vi "UNITEST MAIN v2.0.vi"() -> ()   [LabVIEW 2025] (continued)
            n1370 = property on="Property Node" class="DigNum (strict)"(reference=w2222, "Minimum"=2.0 ("Data Entry Limits:Minimum"), "Maximum"=50.0 ("Data Entry Limits:Maximum"), "Increment"=0.1 ("Data Entry Limits:Increment")) -> (reference out=w2220:refnum<vi>, error out=w2221:errorcluster)  [unwired: 1 in]
            n1371 = call "DATA ENCRYPT STRING FILE WRITE.vi"("error in (no error)"=w2224, "User Action"="User selected 0.3 SSP", "main ref"=w2216) -> ("error out"=w2223:errorcluster)  [unwired: 6 in, 1 out]
            n1372 = Close Reference(reference=w2229, error in (no error)=w2228) -> ()  [unwired: 1 out]
            n1373 = Close Reference(reference=w2230, error in (no error)=w2231) -> ()  [unwired: 1 out]
            n1374 = Close Reference(reference=w2220, error in (no error)=w2221) -> ()  [unwired: 1 out]
          }
        }
      }
      frame "SSP 0.5" {
        n1375 = Unbundle By Name(w2235) -> ("Loading.SSP 0.5"=w2238:refnum<vi>)
        n1376 = property on="Property Node" class="Bool (strict)"(reference=w2238, error in=w2237) -> (reference out=w2240:refnum<vi>, error out=w2239:errorcluster, "Value"=w2236:bool)
        n1377 = Close Reference(reference=w2240, error in (no error)=w2239) -> (error out=w2234:errorcluster)
        n1378 = case shown="True" w2236 {
          tunnel: w2235 -> [_ w2242]
          tunnel: w2234 -> [w2241 w2250]
          tunnel: [w2241 w2249] -> w2233
          frame False {
          }
          frame True {
            w2252 = FALSE ("Value")
            n1379 = Unbundle By Name(w2242) -> ("Loading.Enter the Load  (N)"=w2248:refnum<vi>)
            n1380 = Unbundle By Name(w2242) -> ("Loading.SSP 0.75"=w2258:refnum<vi>)
            n1381 = Unbundle By Name(w2242) -> ("Loading.SSP 0.3"=w2253:refnum<vi>)
            n1382 = property on="Property Node" class="Bool (strict)"(reference=w2253, "Value"=w2252) -> (reference out=w2255:refnum<vi>, error out=w2254:errorcluster)  [unwired: 1 in]
            n1383 = property on="Property Node" class="Bool (strict)"(reference=w2258, "Value"=w2252) -> (reference out=w2256:refnum<vi>, error out=w2257:errorcluster)  [unwired: 1 in]
            n1384 = property on="Property Node" class="DigNum (strict)"(reference=w2248, "Minimum"=2.0 ("Data Entry Limits:Minimum"), "Maximum"=200.0 ("Data Entry Limits:Maximum"), "Increment"=0.1 ("Data Entry Limits:Increment")) -> (reference out=w2246:refnum<vi>, error out=w2247:errorcluster)  [unwired: 1 in]
            n1385 = call "DATA ENCRYPT STRING FILE WRITE.vi"("error in (no error)"=w2250, "User Action"="User selected 0.5 SSP", "main ref"=w2242) -> ("error out"=w2249:errorcluster)  [unwired: 6 in, 1 out]
            n1386 = Close Reference(reference=w2255, error in (no error)=w2254) -> ()  [unwired: 1 out]
            n1387 = Close Reference(reference=w2256, error in (no error)=w2257) -> ()  [unwired: 1 out]
            n1388 = Close Reference(reference=w2246, error in (no error)=w2247) -> ()  [unwired: 1 out]
          }
        }
      }
      frame "SSP 0.75" {
        n1389 = Unbundle By Name(w2261) -> ("Loading.SSP 0.75"=w2264:refnum<vi>)
        n1390 = property on="Property Node" class="Bool (strict)"(reference=w2264, error in=w2263) -> (reference out=w2266:refnum<vi>, error out=w2265:errorcluster, "Value"=w2262:bool)
        n1391 = Close Reference(reference=w2266, error in (no error)=w2265) -> (error out=w2260:errorcluster)
        n1392 = case shown="True" w2262 {
          tunnel: w2261 -> [_ w2268]
          tunnel: w2260 -> [w2267 w2276]
          tunnel: [w2267 w2275] -> w2259
          frame False {
          }
          frame True {
            w2278 = FALSE ("Value")
            n1393 = Unbundle By Name(w2268) -> ("Loading.SSP 0.3"=w2279:refnum<vi>)
            n1394 = Unbundle By Name(w2268) -> ("Loading.SSP 0.5"=w2284:refnum<vi>)
            n1395 = Unbundle By Name(w2268) -> ("Loading.Enter the Load  (N)"=w2274:refnum<vi>)
            n1396 = property on="Property Node" class="Bool (strict)"(reference=w2279, "Value"=w2278) -> (reference out=w2281:refnum<vi>, error out=w2280:errorcluster)  [unwired: 1 in]
            n1397 = property on="Property Node" class="Bool (strict)"(reference=w2284, "Value"=w2278) -> (reference out=w2282:refnum<vi>, error out=w2283:errorcluster)  [unwired: 1 in]
            n1398 = property on="Property Node" class="DigNum (strict)"(reference=w2274, "Minimum"=200.0 ("Data Entry Limits:Minimum"), "Maximum"=500.0 ("Data Entry Limits:Maximum"), "Increment"=0.1 ("Data Entry Limits:Increment")) -> (reference out=w2272:refnum<vi>, error out=w2273:errorcluster)  [unwired: 1 in]
            n1399 = call "DATA ENCRYPT STRING FILE WRITE.vi"("error in (no error)"=w2276, "User Action"="User selected 0.75 SSP", "main ref"=w2268) -> ("error out"=w2275:errorcluster)  [unwired: 6 in, 1 out]
            n1400 = Close Reference(reference=w2281, error in (no error)=w2280) -> ()  [unwired: 1 out]
            n1401 = Close Reference(reference=w2282, error in (no error)=w2283) -> ()  [unwired: 1 out]
            n1402 = Close Reference(reference=w2272, error in (no error)=w2273) -> ()  [unwired: 1 out]
          }
        }
      }
      frame "LHBack" {
        # "Back to Configure"
        n1403 = Unbundle By Name(w2286) -> ("Main Home Screen.GUI"=w2295:refnum<vi>)
        n1404 = Unbundle By Name(w2286) -> ("Main Home Screen.MainPage"=w2291:refnum<vi>)
        n1405 = Unbundle By Name(w2286) -> ("Loading.LHBack"=w2289:refnum<vi>)
        n1406 = property on="Property Node" class="TabCtl (strict)"(reference=w2291, "Value"=T16."HOME") -> (reference out=w2293:refnum<vi>, error out=w2292:errorcluster)  [unwired: 1 in]
        n1407 = property on="Property Node" class="Bool (strict)"(reference=w2289, "Value"=FALSE) -> (reference out=w2287:refnum<vi>, error out=w2288:errorcluster)  [unwired: 1 in]
        n1408 = property on="Property Node" class="TabCtl (strict)"(reference=w2295, "Value"=T15."Setup") -> (reference out=w2297:refnum<vi>, error out=w2296:errorcluster)  [unwired: 1 in]
        n1409 = Close Reference(reference=w2293, error in (no error)=w2292) -> ()  [unwired: 1 out]
        n1410 = Close Reference(reference=w2287, error in (no error)=w2288) -> ()  [unwired: 1 out]
        n1411 = Close Reference(reference=w2297, error in (no error)=w2296) -> ()  [unwired: 1 out]
        n1412 = call "DATA ENCRYPT STRING FILE WRITE.vi"("error in (no error)"=w2298, "User Action"="User selected Back to Configure", "main ref"=w2286) -> ("error out"=w2299:errorcluster)  [unwired: 6 in, 1 out]
      }
      frame "MMBack" {
        # "Back to Configure"
        n1413 = Unbundle By Name(w2301) -> ("Motion Module.MMBack"=w2305:refnum<vi>)
        n1414 = Unbundle By Name(w2301) -> ("Main Home Screen.GUI"=w2311:refnum<vi>)
        n1415 = Unbundle By Name(w2301) -> ("Main Home Screen.MainPage"=w2307:refnum<vi>)
        n1416 = property on="Property Node" class="Bool (strict)"(reference=w2305, "Value"=FALSE) -> (reference out=w2303:refnum<vi>, error out=w2304:errorcluster)  [unwired: 1 in]
        n1417 = property on="Property Node" class="TabCtl (strict)"(reference=w2307, "Value"=T16."HOME") -> (reference out=w2309:refnum<vi>, error out=w2308:errorcluster)  [unwired: 1 in]
        n1418 = property on="Property Node" class="TabCtl (strict)"(reference=w2311, "Value"=T15."Load Head") -> (reference out=w2313:refnum<vi>, error out=w2312:errorcluster)  [unwired: 1 in]
        n1419 = Close Reference(reference=w2303, error in (no error)=w2304) -> ()  [unwired: 1 out]
        n1420 = Close Reference(reference=w2309, error in (no error)=w2308) -> ()  [unwired: 1 out]
        n1421 = Close Reference(reference=w2313, error in (no error)=w2312) -> ()  [unwired: 1 out]
        n1422 = call "DATA ENCRYPT STRING FILE WRITE.vi"("error in (no error)"=w2314, "User Action"="User selected Back to Load Selection", "main ref"=w2301) -> ("error out"=w2315:errorcluster)  [unwired: 6 in, 1 out]
      }
      frame "LHNext" {
        w2351 = FALSE ("Visible")
        n1423 = Unbundle By Name(w2317) -> ("Motion Module.HomeRot"=w2357:refnum<vi>)
        n1424 = Unbundle By Name(w2317) -> ("Motion Module.HomeScratch"=w2352:refnum<vi>)
        n1425 = Unbundle By Name(w2317) -> ("Motion Module.PlaceModule"=w2350:refnum<vi>)
        n1426 = Unbundle By Name(w2317) -> ("Motion Module.Motion Mode:"=w2343:refnum<vi>)
        n1427 = Unbundle By Name(w2317) -> ("Motion Module.Motion Direction:  3"=w2342:refnum<vi>)
        n1428 = Unbundle By Name(w2317) -> ("Motion Module.Wear Track Diameter (mm)"=w2336:refnum<vi>)
        n1429 = Unbundle By Name(w2317) -> ("Motion Module.Set WTD"=w2333:refnum<vi>)
        n1430 = Unbundle By Name(w2317) -> ("Motion Module.Rotary Module Selection"=w2327:refnum<vi>)
        n1431 = call "DATA ENCRYPT STRING FILE WRITE.vi"("error in (no error)"=w2366, "User Action"="User selected Select Module", "main ref"=w2317) -> ("error out"=w2330:errorcluster)  [unwired: 6 in, 1 out]
        n1432 = property on="Property Node" class="TabCtl (strict)"(reference=w2327, "Visible"=FALSE) -> (reference out=w2326:refnum<vi>, error out=w2328:errorcluster)  [unwired: 1 in]
        n1433 = property on="Property Node" class="Bool (strict)"(reference=w2357, error in=w2330, "Visible"=w2351) -> (reference out=w2355:refnum<vi>, error out=w2356:errorcluster)
        n1434 = property on="Property Node" class="Bool (strict)"(reference=w2352, error in=w2330, "Visible"=w2351) -> (reference out=w2354:refnum<vi>, error out=w2353:errorcluster)
        n1435 = property on="Property Node" class="Bool (strict)"(reference=w2350, error in=w2330, "Visible"=TRUE) -> (reference out=w2348:refnum<vi>, error out=w2349:errorcluster)
        n1436 = property on="Property Node" class="Ring (strict)"(reference=w2343, error in=w2330, "Visible"=FALSE) -> (reference out=w2345:refnum<vi>, error out=w2344:errorcluster)
        n1437 = property on="Property Node" class="Ring (strict)"(reference=w2342, error in=w2330, "Visible"=FALSE) -> (reference out=w2339:refnum<vi>, error out=w2341:errorcluster)
        n1438 = property on="Property Node" class="DigNum (strict)"(reference=w2336, "Visible"=FALSE) -> (reference out=w2335:refnum<vi>, error out=w2337:errorcluster)  [unwired: 1 in]
        n1439 = property on="Property Node" class="Bool (strict)"(reference=w2333, "Visible"=FALSE) -> (reference out=w2334:refnum<vi>, error out=w2332:errorcluster)  [unwired: 1 in]
        n1440 = Close Reference(reference=w2355, error in (no error)=w2356) -> ()  [unwired: 1 out]
        n1441 = Close Reference(reference=w2354, error in (no error)=w2353) -> ()  [unwired: 1 out]
        n1442 = Close Reference(reference=w2348, error in (no error)=w2349) -> ()  [unwired: 1 out]
        n1443 = Close Reference(reference=w2345, error in (no error)=w2344) -> ()  [unwired: 1 out]
        n1444 = Close Reference(reference=w2339, error in (no error)=w2341) -> ()  [unwired: 1 out]
        n1445 = Close Reference(reference=w2335, error in (no error)=w2337) -> ()  [unwired: 1 out]
        n1446 = Close Reference(reference=w2326, error in (no error)=w2328) -> ()  [unwired: 1 out]
        n1447 = Close Reference(reference=w2334, error in (no error)=w2332) -> ()  [unwired: 1 out]
        n1448 = Unbundle By Name(w2317) -> ("Motion Module.M3 Image"=w2325:refnum<vi>)
        n1449 = Unbundle By Name(w2317) -> ("Main Home Screen.GUI"=w2363:refnum<vi>)
        n1450 = Unbundle By Name(w2317) -> ("Main Home Screen.MainPage"=w2359:refnum<vi>)
        n1451 = Unbundle By Name(w2317) -> ("Loading.LHNext"=w2321:refnum<vi>)
        n1452 = property on="Property Node" class="TabCtl (strict)"(reference=w2325, "Value"=enum32{"Page 1", "Page 2"}."Page 2") -> (reference out=w2323:refnum<vi>, error out=w2324:errorcluster)  [unwired: 1 in]
        n1453 = property on="Property Node" class="TabCtl (strict)"(reference=w2359, "Value"=T16."HOME") -> (reference out=w2361:refnum<vi>, error out=w2360:errorcluster)  [unwired: 1 in]
        n1454 = property on="Property Node" class="TabCtl (strict)"(reference=w2363, "Value"=T15."Motion Module") -> (reference out=w2365:refnum<vi>, error out=w2364:errorcluster)  [unwired: 1 in]
        n1455 = property on="Property Node" class="Bool (strict)"(reference=w2321, "Value"=FALSE ("Visible")) -> (reference out=w2318:refnum<vi>, error out=w2320:errorcluster)  [unwired: 1 in]
        n1456 = Close Reference(reference=w2323, error in (no error)=w2324) -> ()  [unwired: 1 out]
        n1457 = Close Reference(reference=w2318, error in (no error)=w2320) -> ()  [unwired: 1 out]
        n1458 = Close Reference(reference=w2361, error in (no error)=w2360) -> ()  [unwired: 1 out]
        n1459 = Close Reference(reference=w2365, error in (no error)=w2364) -> ()  [unwired: 1 out]
      }
      frame "Rot Ver" {
        n1460 = call "Rotory Module Selection.vi"("error in (no error)"=w2370, "Data Cluster"=w2368) -> ("error out"=w2369:errorcluster)  [unwired: 9 in]
      }
      frame "Scratch" {
        n1461 = call "Scratch Module Selection.vi"("error in (no error)"=w2373, "Data Cluster"=w2371) -> ("error out"=w2372:errorcluster)  [unwired: 9 in]
      }
      frame "Traction" {
        n1462 = call "TractionModule Selection.vi"("error in (no error)"=w2376, "Data Cluster"=w2374) -> ("error out"=w2375:errorcluster)  [unwired: 9 in]
      }
      frame "Motion Mode:" {
        n1463 = Unbundle By Name(w2377) -> ("Motion Module.Motion Mode:"=w2379:refnum<vi>)
        n1464 = property on="Property Node" class="Ring (strict)"(reference=w2379) -> (reference out=w2381:refnum<vi>, error out=w2380:errorcluster, "Value"=w2378:u16)  [unwired: 1 in]
        n1465 = Close Reference(reference=w2381, error in (no error)=w2380) -> ()  [unwired: 1 out]
        n1466 = case shown="3" w2378 {
          tunnel: w2383 -> [w2400 w2417 w2434 w2451]
          tunnel: [w2399 w2416 w2433 w2450] -> w2382
          tunnel: w2377 -> [w2398 w2415 w2432 w2449]
          tunnel: w2377 -> [w2384 w2402 w2418 w2435]
          frame 0, Default {
            n1467 = Unbundle By Name(w2384) -> ("Motion Module.Rotary Module Selection"=w2394:refnum<vi>)
            n1468 = Unbundle By Name(w2384) -> ("Motion Module.Motion Direction:  3"=w2392:refnum<vi>)
            n1469 = Unbundle By Name(w2384) -> ("Main Screen.Angle (Deg)"=w2386:refnum<vi>)
            n1470 = property on="Property Node" class="TabCtl (strict)"(reference=w2394, "Value"=T18."Uniform Rotation") -> (reference out=w2396:refnum<vi>, error out=w2395:errorcluster)  [unwired: 1 in]
            n1471 = property on="Property Node" class="DigNum (strict)"(reference=w2386, "DisabledEnum"=T31."Disabled and Grayed Out" ("Disabled")) -> (reference out=w2388:refnum<vi>, error out=w2387:errorcluster)  [unwired: 1 in]
            n1472 = property on="Property Node" class="Ring (strict)"(reference=w2392, "Visible"=TRUE) -> (reference out=w2390:refnum<vi>, error out=w2391:errorcluster)  [unwired: 1 in]
            n1473 = Close Reference(reference=w2396, error in (no error)=w2395) -> ()  [unwired: 1 out]
            n1474 = Close Reference(reference=w2388, error in (no error)=w2387) -> ()  [unwired: 1 out]
            n1475 = Close Reference(reference=w2390, error in (no error)=w2391) -> ()  [unwired: 1 out]
            n1476 = call "DATA ENCRYPT STRING FILE WRITE.vi"("error in (no error)"=w2400, "User Action"="User Selected Uniform Rotation", "main ref"=w2398) -> ("error out"=w2399:errorcluster)  [unwired: 6 in, 1 out]
          }
          frame 1 {
            n1477 = Unbundle By Name(w2402) -> ("Motion Module.Rotary Module Selection"=w2411:refnum<vi>)
            n1478 = Unbundle By Name(w2402) -> ("Motion Module.Motion Direction:  3"=w2409:refnum<vi>)
            n1479 = Unbundle By Name(w2402) -> ("Main Screen.Angle (Deg)"=w2403:refnum<vi>)
            n1480 = property on="Property Node" class="TabCtl (strict)"(reference=w2411, "Value"=T18."Angular Oscillation") -> (reference out=w2413:refnum<vi>, error out=w2412:errorcluster)  [unwired: 1 in]
            n1481 = property on="Property Node" class="DigNum (strict)"(reference=w2403, "DisabledEnum"=T31."Enabled" ("Disabled")) -> (reference out=w2405:refnum<vi>, error out=w2404:errorcluster)  [unwired: 1 in]
            n1482 = property on="Property Node" class="Ring (strict)"(reference=w2409, "Visible"=FALSE) -> (reference out=w2407:refnum<vi>, error out=w2408:errorcluster)  [unwired: 1 in]
            n1483 = Close Reference(reference=w2413, error in (no error)=w2412) -> ()  [unwired: 1 out]
            n1484 = Close Reference(reference=w2407, error in (no error)=w2408) -> ()  [unwired: 1 out]
            n1485 = Close Reference(reference=w2405, error in (no error)=w2404) -> ()  [unwired: 1 out]
            n1486 = call "DATA ENCRYPT STRING FILE WRITE.vi"("error in (no error)"=w2417, "User Action"="User Selected Angular Oscillation", "main ref"=w2415) -> ("error out"=w2416:errorcluster)  [unwired: 6 in, 1 out]
          }
          frame 2 {
            n1487 = Unbundle By Name(w2418) -> ("Motion Module.Rotary Module Selection"=w2428:refnum<vi>)
            n1488 = Unbundle By Name(w2418) -> ("Motion Module.Motion Direction:  3"=w2426:refnum<vi>)
            n1489 = Unbundle By Name(w2418) -> ("Main Screen.Angle (Deg)"=w2420:refnum<vi>)
            n1490 = property on="Property Node" class="DigNum (strict)"(reference=w2420, "DisabledEnum"=T31."Disabled and Grayed Out" ("Disabled")) -> (reference out=w2422:refnum<vi>, error out=w2421:errorcluster)  [unwired: 1 in]
            n1491 = property on="Property Node" class="TabCtl (strict)"(reference=w2428, "Value"=T18."Speed Ramp") -> (reference out=w2430:refnum<vi>, error out=w2429:errorcluster)  [unwired: 1 in]
            n1492 = property on="Property Node" class="Ring (strict)"(reference=w2426, "Visible"=TRUE) -> (reference out=w2424:refnum<vi>, error out=w2425:errorcluster)  [unwired: 1 in]
            n1493 = Close Reference(reference=w2422, error in (no error)=w2421) -> ()  [unwired: 1 out]
            n1494 = Close Reference(reference=w2430, error in (no error)=w2429) -> ()  [unwired: 1 out]
            n1495 = Close Reference(reference=w2424, error in (no error)=w2425) -> ()  [unwired: 1 out]
            n1496 = call "DATA ENCRYPT STRING FILE WRITE.vi"("error in (no error)"=w2434, "User Action"="User Selected Ramp Mode", "main ref"=w2432) -> ("error out"=w2433:errorcluster)  [unwired: 6 in, 1 out]
          }
          frame 3 {
            n1497 = Unbundle By Name(w2435) -> ("Motion Module.Rotary Module Selection"=w2445:refnum<vi>)
            n1498 = Unbundle By Name(w2435) -> ("Motion Module.Motion Direction:  3"=w2443:refnum<vi>)
            n1499 = Unbundle By Name(w2435) -> ("Main Screen.Angle (Deg)"=w2437:refnum<vi>)
            n1500 = property on="Property Node" class="TabCtl (strict)"(reference=w2445, "Value"=T18."Speed Step") -> (reference out=w2447:refnum<vi>, error out=w2446:errorcluster)  [unwired: 1 in]
            n1501 = property on="Property Node" class="DigNum (strict)"(reference=w2437, "DisabledEnum"=T31."Disabled and Grayed Out" ("Disabled")) -> (reference out=w2439:refnum<vi>, error out=w2438:errorcluster)  [unwired: 1 in]
            n1502 = property on="Property Node" class="Ring (strict)"(reference=w2443, "Visible"=FALSE) -> (reference out=w2441:refnum<vi>, error out=w2442:errorcluster)  [unwired: 1 in]
            n1503 = Close Reference(reference=w2447, error in (no error)=w2446) -> ()  [unwired: 1 out]
            n1504 = Close Reference(reference=w2439, error in (no error)=w2438) -> ()  [unwired: 1 out]
            n1505 = Close Reference(reference=w2441, error in (no error)=w2442) -> ()  [unwired: 1 out]
            n1506 = call "DATA ENCRYPT STRING FILE WRITE.vi"("error in (no error)"=w2451, "User Action"="User Selected Step Mode", "main ref"=w2449) -> ("error out"=w2450:errorcluster)  [unwired: 6 in, 1 out]
          }
        }
      }
      frame "MMNext" {
        n1507 = Unbundle By Name(w2452) -> ("Motion Module.MMNext"=w2457:refnum<vi>)
        n1508 = Unbundle By Name(w2452) -> ("Motion Module.MMNext"=w2464:refnum<vi>)
        n1509 = Unbundle By Name(w2452) -> ("Main Home Screen.GUI"=w2466:refnum<vi>)
        n1510 = property on="Property Node" class="Bool (strict)"(reference=w2457, "Value"=FALSE ("Visible")) -> (reference out=w2454:refnum<vi>, error out=w2456:errorcluster)  [unwired: 1 in]
        n1511 = property on="Property Node" class="TabCtl (strict)"(reference=w2466, "Value"=T15."Environment") -> (reference out=w2468:refnum<vi>, error out=w2467:errorcluster)  [unwired: 1 in]
        n1512 = property on="Property Node" class="Bool (strict)"(reference=w2464, "Value"=FALSE) -> (reference out=w2462:refnum<vi>, error out=w2463:errorcluster)  [unwired: 1 in]
        n1513 = Close Reference(reference=w2454, error in (no error)=w2456) -> ()  [unwired: 1 out]
        n1514 = Close Reference(reference=w2462, error in (no error)=w2463) -> ()  [unwired: 1 out]
        n1515 = Close Reference(reference=w2468, error in (no error)=w2467) -> ()  [unwired: 1 out]
        n1516 = call "DATA ENCRYPT STRING FILE WRITE.vi"("error in (no error)"=w2459, "User Action"="User Selected SetUp Module", "main ref"=w2452) -> ("error out"=w2458:errorcluster)  [unwired: 6 in, 1 out]
        n1517 = call "Main Screen Tab Visible.vi"("error in (no error)"=w2458, "main ref"=w2452) -> ("error out"=w2453:errorcluster)  [unwired: 9 in]
      }
      frame "APBack" {
        n1518 = Unbundle By Name(w2469) -> ("Environmental control.APBack"=w2476:refnum<vi>)
        n1519 = Unbundle By Name(w2469) -> ("Main Home Screen.GUI"=w2478:refnum<vi>)
        n1520 = property on="Property Node" class="TabCtl (strict)"(reference=w2478, "Value"=T15."Motion Module") -> (reference out=w2480:refnum<vi>, error out=w2479:errorcluster)  [unwired: 1 in]
        n1521 = property on="Property Node" class="Bool (strict)"(reference=w2476, "Value"=FALSE) -> (reference out=w2474:refnum<vi>, error out=w2475:errorcluster)  [unwired: 1 in]
        n1522 = Close Reference(reference=w2474, error in (no error)=w2475) -> ()  [unwired: 1 out]
        n1523 = Close Reference(reference=w2480, error in (no error)=w2479) -> ()  [unwired: 1 out]
        n1524 = call "DATA ENCRYPT STRING FILE WRITE.vi"("error in (no error)"=w2471, "User Action"="User Selected Back to Module", "main ref"=w2469) -> ("error out"=w2470:errorcluster)  [unwired: 6 in, 1 out]
      }
      frame "SNext" {
        n1525 = Unbundle By Name(w2482) -> ("Environmental control.Acoustic Emission 3"=w2486:refnum<vi>)
        n1526 = property on="Property Node" class="Bool (strict)"(reference=w2486) -> (reference out=w2484:refnum<vi>, error out=w2485:errorcluster, "Value"=w2481:bool)  [unwired: 1 in]
        n1527 = Close Reference(reference=w2484, error in (no error)=w2485) -> ()  [unwired: 1 out]
        n1528 = case shown="True" w2481 {
          tunnel: w2488 -> [w2491 w2495]
          tunnel: [w2491 w2492] -> w2483
          tunnel: w2482 -> [_ w2493]
          frame False {
          }
          frame True {
            n1529 = call "Acq Gain Selection.vi"("error in (no error)"=w2495, "Data Cluster"=w2493) -> ("error out"=w2494:errorcluster)  [unwired: 9 in]
            n1530 = call <vilib>:"Clear Errors.vi"("error in (no error)"=w2494) -> ("error out"=w2492:errorcluster)  [unwired: 5 in, 1 out]
          }
        }
        n1531 = call "Init Before Main Screen.vi"("error in (no error)"=w2483, "Data Cluster"=w2482) -> ("error out"=w2487:errorcluster)  [unwired: 9 in]
        n1532 = call "DATA ENCRYPT STRING FILE WRITE.vi"("error in (no error)"=w2487, "User Action"="User Pressed Setup", "main ref"=w2482) -> ("error out"=w2489:errorcluster)  [unwired: 6 in, 1 out]
      }
      frame "Enable Platform" {
        n1533 = call "Reinitialise Load cell after Error.vi"("error in (no error)"=w2499, "main ref"=w2496) -> ("error out"=w2497:errorcluster)  [unwired: 9 in]
        n1534 = Unbundle By Name(w2496) -> ("Platform Settings.Enable Platform"=w2523:refnum<vi>)
        n1535 = Bundle By Name(cluster=T9 {"Sequence ID"=0, "Mode Command"=0, "Distance"=0.0, "SPEED"=0.0, "Reserved"=0.0, "SPARE 1"=0, "SPARE 2"=0, "SPARE 3"=0, "SPARE 4"=0, "SPARE 5"=0, "SPARE 6"=0, "SPARE 7"=0, "SPARE 8"=0, "SPARE 9"=0, "SPARE 10"=0, "SPARE 11"=0, "SPARE 12"=0, "SPARE 13"=0, "SPARE 14"=0, "SPARE 15"=0, "SPARE 16"=0, "SPARE 17"=0} ("Value"), "Mode Command"=u8 1, "Distance"=sgl 0.0, "SPEED"=sgl 0.0, "Sequence ID"=u16 0) -> (w2508:T9)
        n1536 = Unbundle By Name(w2496) -> ("Heave AND Surge.UPLINK HEAVE"=w2501:refnum<vi>)
        n1537 = property on="Property Node" class="Bool (strict)"(reference=w2523, "Value"=FALSE) -> (reference out=w2521:refnum<vi>, error out=w2522:errorcluster)  [unwired: 1 in]
        n1538 = property on="Property Node" class="Clust (strict)"(reference=w2501, error in=w2497, "Value"=w2508) -> (reference out=w2507:refnum<vi>, error out=w2506:errorcluster)
        n1539 = Close Reference(reference=w2521, error in (no error)=w2522) -> ()  [unwired: 1 out]
        n1540 = Close Reference(reference=w2507, error in (no error)=w2506) -> (error out=w2498:errorcluster)
        n1541 = call "DATA ENCRYPT STRING FILE WRITE.vi"("error in (no error)"=w2498, "User Action"="User Pressed Enable Platform", "main ref"=w2496) -> ("error out"=w2510:errorcluster)  [unwired: 6 in, 1 out]
        n1542 = call "HEAVE WRITE FGV.vi"("Enum - Menu"=Heave_Write_enum."WRITE", "error in (no error)"=w2510, "main ref"=w2496) -> ("error out"=w2513:errorcluster)  [unwired: 8 in]
        n1543 = call "TRACTION HOME.vi"("error in (no error)"=w2510, "Data Cluster"=w2496) -> ("error out"=→"error out":errorcluster)  [unwired: 9 in]
        n1544 = Unbundle By Name(w2496) -> ("Heave AND Surge.Read Heave Temp"=w2517:refnum<vi>)
        n1545 = property on="Property Node" class="Bool (strict)"(reference=w2517, error in=w2513, "Value"=TRUE) -> (reference out=w2515:refnum<vi>, error out=w2516:errorcluster)
        n1546 = Close Reference(reference=w2515, error in (no error)=w2516) -> (error out=w2512:errorcluster)
        "HEAVE ENABLE" <- TRUE ("HEAVE ENABLE")
      }
      frame "Heave Up main" {
        n1547 = Unbundle By Name(w2524) -> ("Platform Settings.Heave Up main"=w2534:refnum<vi>)
        n1548 = call "Heave Up Main.vi"("error in (no error)"=w2526, "main ref"=w2524) -> ("error out"=w2525:errorcluster)  [unwired: 9 in]
        n1549 = property on="Property Node" class="Bool (strict)"(reference=w2534, "Value"=FALSE) -> (reference out=w2532:refnum<vi>, error out=w2533:errorcluster)  [unwired: 1 in]
        n1550 = Close Reference(reference=w2532, error in (no error)=w2533) -> ()  [unwired: 1 out]
        n1551 = call "DATA ENCRYPT STRING FILE WRITE.vi"("error in (no error)"=w2525, "User Action"="User Pressed Heave UP", "main ref"=w2524) -> ("error out"=w2529:errorcluster)  [unwired: 6 in, 1 out]
        n1552 = call "HEAVE WRITE FGV.vi"("Enum - Menu"=Heave_Write_enum."WRITE", "error in (no error)"=w2529, "main ref"=w2524) -> ("error out"=w2528:errorcluster)  [unwired: 8 in]
      }
      frame "Heave Up MM" {
        n1553 = Unbundle By Name(w2535) -> ("Motion Module.Heave Up MM"=w2545:refnum<vi>)
        n1554 = call "Heave Up Motion Module.vi"("error in (no error)"=w2537, "main ref"=w2535) -> ("error out"=w2536:errorcluster)  [unwired: 9 in]
        n1555 = property on="Property Node" class="Bool (strict)"(reference=w2545, "Value"=FALSE) -> (reference out=w2543:refnum<vi>, error out=w2544:errorcluster)  [unwired: 1 in]
        n1556 = Close Reference(reference=w2543, error in (no error)=w2544) -> ()  [unwired: 1 out]
        n1557 = call "DATA ENCRYPT STRING FILE WRITE.vi"("error in (no error)"=w2536, "User Action"="User Pressed Heave UP in Motion Module", "main ref"=w2535) -> ("error out"=w2540:errorcluster)  [unwired: 6 in, 1 out]
        n1558 = call "HEAVE WRITE FGV.vi"("Enum - Menu"=Heave_Write_enum."WRITE", "error in (no error)"=w2540, "main ref"=w2535) -> ("error out"=w2539:errorcluster)  [unwired: 8 in]
      }
      frame "Heave Down Main" {
        n1559 = call "Heave Down Main.vi"("error in (no error)"=w2548, "main ref"=w2546) -> ("error out"=w2547:errorcluster)  [unwired: 9 in]
        n1560 = Unbundle By Name(w2546) -> ("Platform Settings.Heave Down Main"=w2556:refnum<vi>)
        n1561 = property on="Property Node" class="Bool (strict)"(reference=w2556, "Value"=FALSE) -> (reference out=w2554:refnum<vi>, error out=w2555:errorcluster)  [unwired: 1 in]
        n1562 = Close Reference(reference=w2554, error in (no error)=w2555) -> ()  [unwired: 1 out]
        n1563 = call "DATA ENCRYPT STRING FILE WRITE.vi"("error in (no error)"=w2547, "User Action"="User Pressed Heave DOWN", "main ref"=w2546) -> ("error out"=w2551:errorcluster)  [unwired: 6 in, 1 out]
        n1564 = call "HEAVE WRITE FGV.vi"("Enum - Menu"=Heave_Write_enum."WRITE", "error in (no error)"=w2551, "main ref"=w2546) -> ("error out"=w2550:errorcluster)  [unwired: 8 in]
      }
      frame "Heave Down MM" {
        n1565 = call "Heave Down Motion Module.vi"("error in (no error)"=w2559, "main ref"=w2557) -> ("error out"=w2558:errorcluster)  [unwired: 9 in]
        n1566 = Unbundle By Name(w2557) -> ("Motion Module.Heave Down MM"=w2567:refnum<vi>)
        n1567 = property on="Property Node" class="Bool (strict)"(reference=w2567, "Value"=FALSE) -> (reference out=w2565:refnum<vi>, error out=w2566:errorcluster)  [unwired: 1 in]
        n1568 = Close Reference(reference=w2565, error in (no error)=w2566) -> ()  [unwired: 1 out]
        n1569 = call "DATA ENCRYPT STRING FILE WRITE.vi"("error in (no error)"=w2558, "User Action"="User Pressed Heave DOWN in Motion Module", "main ref"=w2557) -> ("error out"=w2562:errorcluster)  [unwired: 6 in, 1 out]
        n1570 = call "HEAVE WRITE FGV.vi"("Enum - Menu"=Heave_Write_enum."WRITE", "error in (no error)"=w2562, "main ref"=w2557) -> ("error out"=w2561:errorcluster)  [unwired: 8 in]
      }
      frame "Surge Backward Main" {
        n1571 = Unbundle By Name(w2568) -> ("Platform Settings.Surge Backward Main"=w2578:refnum<vi>)
        n1572 = call "Surge Backward Main.vi"("error in (no error)"=w2570, "main ref"=w2568) -> ("error out"=w2569:errorcluster)  [unwired: 9 in]
        n1573 = property on="Property Node" class="Bool (strict)"(reference=w2578, "Value"=FALSE) -> (reference out=w2576:refnum<vi>, error out=w2577:errorcluster)  [unwired: 1 in]
        n1574 = Close Reference(reference=w2576, error in (no error)=w2577) -> ()  [unwired: 1 out]
        n1575 = call "DATA ENCRYPT STRING FILE WRITE.vi"("error in (no error)"=w2569, "User Action"="User Pressed Surge Backward", "main ref"=w2568) -> ("error out"=w2573:errorcluster)  [unwired: 6 in, 1 out]
        n1576 = call "HEAVE WRITE FGV.vi"("Enum - Menu"=Heave_Write_enum."WRITE", "error in (no error)"=w2573, "main ref"=w2568) -> ("error out"=w2572:errorcluster)  [unwired: 8 in]
      }
      frame "Surge Backward MM" {
        n1577 = Unbundle By Name(w2579) -> ("Motion Module.Surge Backward MM"=w2589:refnum<vi>)
        n1578 = call "Surge Backward MM.vi"("error in (no error)"=w2581, "main ref"=w2579) -> ("error out"=w2580:errorcluster)  [unwired: 9 in]
        n1579 = property on="Property Node" class="Bool (strict)"(reference=w2589, "Value"=FALSE) -> (reference out=w2587:refnum<vi>, error out=w2588:errorcluster)  [unwired: 1 in]
        n1580 = Close Reference(reference=w2587, error in (no error)=w2588) -> ()  [unwired: 1 out]
        n1581 = call "DATA ENCRYPT STRING FILE WRITE.vi"("error in (no error)"=w2580, "User Action"="User Pressed Surge Backward in Motion Module", "main ref"=w2579) -> ("error out"=w2584:errorcluster)  [unwired: 6 in, 1 out]
        n1582 = call "HEAVE WRITE FGV.vi"("Enum - Menu"=Heave_Write_enum."WRITE", "error in (no error)"=w2584, "main ref"=w2579) -> ("error out"=w2583:errorcluster)  [unwired: 8 in]
      }
      frame "Surge Forward Main" {
        n1583 = Unbundle By Name(w2590) -> ("Platform Settings.Surge Forward Main"=w2600:refnum<vi>)
        n1584 = call "Surge Forward Main.vi"("error in (no error)"=w2592, "main ref"=w2590) -> ("error out"=w2591:errorcluster)  [unwired: 9 in]
        n1585 = property on="Property Node" class="Bool (strict)"(reference=w2600, "Value"=FALSE) -> (reference out=w2598:refnum<vi>, error out=w2599:errorcluster)  [unwired: 1 in]
        n1586 = Close Reference(reference=w2598, error in (no error)=w2599) -> ()  [unwired: 1 out]
        n1587 = call "DATA ENCRYPT STRING FILE WRITE.vi"("error in (no error)"=w2591, "User Action"="User Pressed Surge Forward", "main ref"=w2590) -> ("error out"=w2595:errorcluster)  [unwired: 6 in, 1 out]
        n1588 = call "HEAVE WRITE FGV.vi"("Enum - Menu"=Heave_Write_enum."WRITE", "error in (no error)"=w2595, "main ref"=w2590) -> ("error out"=w2594:errorcluster)  [unwired: 8 in]
      }
      frame "Surge Forward MM" {
        n1589 = Unbundle By Name(w2601) -> ("Motion Module.Surge Forward MM"=w2611:refnum<vi>)
        n1590 = call "Surge Forward MM.vi"("error in (no error)"=w2603, "main ref"=w2601) -> ("error out"=w2602:errorcluster)  [unwired: 9 in]
        n1591 = property on="Property Node" class="Bool (strict)"(reference=w2611, "Value"=FALSE) -> (reference out=w2609:refnum<vi>, error out=w2610:errorcluster)  [unwired: 1 in]
        n1592 = Close Reference(reference=w2609, error in (no error)=w2610) -> ()  [unwired: 1 out]
        n1593 = call "DATA ENCRYPT STRING FILE WRITE.vi"("error in (no error)"=w2602, "User Action"="User Pressed Surge Forward in Motion Module", "main ref"=w2601) -> ("error out"=w2606:errorcluster)  [unwired: 6 in, 1 out]
        n1594 = call "HEAVE WRITE FGV.vi"("Enum - Menu"=Heave_Write_enum."WRITE", "error in (no error)"=w2606, "main ref"=w2601) -> ("error out"=w2605:errorcluster)  [unwired: 8 in]
      }
      frame "Sway Left Main" {
        n1595 = call "Sway Left Main.vi"("error in (no error)"=w2615, "main ref"=w2613) -> ("error out"=w2614:errorcluster)  [unwired: 9 in]
        n1596 = Unbundle By Name(w2613) -> ("Platform Settings.Sway Left Main"=w2622:refnum<vi>)
        n1597 = property on="Property Node" class="Bool (strict)"(reference=w2622, "Value"=FALSE) -> (reference out=w2620:refnum<vi>, error out=w2621:errorcluster)  [unwired: 1 in]
        n1598 = Close Reference(reference=w2620, error in (no error)=w2621) -> ()  [unwired: 1 out]
        n1599 = call "DATA ENCRYPT STRING FILE WRITE.vi"("error in (no error)"=w2614, "User Action"="User Pressed Sway Left ", "main ref"=w2613) -> ("error out"=w2617:errorcluster)  [unwired: 6 in, 1 out]
        n1600 = call "SWAY WRITE FGV.vi"("Enum - Menu"=Sway_Write_enum."WRITE", "error in (no error)"=w2617, "main ref"=w2613) -> ("error out"=w2616:errorcluster)  [unwired: 8 in]
      }
      frame "Sway Left MM" {
        n1601 = call "Sway Left MM.vi"("error in (no error)"=w2626, "main ref"=w2624) -> ("error out"=w2625:errorcluster)  [unwired: 9 in]
        n1602 = Unbundle By Name(w2624) -> ("Motion Module.Sway Left MM"=w2633:refnum<vi>)
        n1603 = property on="Property Node" class="Bool (strict)"(reference=w2633, "Value"=FALSE) -> (reference out=w2631:refnum<vi>, error out=w2632:errorcluster)  [unwired: 1 in]
        n1604 = Close Reference(reference=w2631, error in (no error)=w2632) -> ()  [unwired: 1 out]
        n1605 = call "DATA ENCRYPT STRING FILE WRITE.vi"("error in (no error)"=w2625, "User Action"="User Pressed Sway Left in MM", "main ref"=w2624) -> ("error out"=w2628:errorcluster)  [unwired: 6 in, 1 out]
        n1606 = call "SWAY WRITE FGV.vi"("Enum - Menu"=Sway_Write_enum."WRITE", "error in (no error)"=w2628, "main ref"=w2624) -> ("error out"=w2627:errorcluster)  [unwired: 8 in]
      }
      frame "Sway Right MM" {
        n1607 = call "Sway Right MM.vi"("error in (no error)"=w2637, "main ref"=w2635) -> ("error out"=w2636:errorcluster)  [unwired: 9 in]
        n1608 = Unbundle By Name(w2635) -> ("Motion Module.Sway Right MM"=w2644:refnum<vi>)
        n1609 = property on="Property Node" class="Bool (strict)"(reference=w2644, "Value"=FALSE) -> (reference out=w2642:refnum<vi>, error out=w2643:errorcluster)  [unwired: 1 in]
        n1610 = Close Reference(reference=w2642, error in (no error)=w2643) -> ()  [unwired: 1 out]
        n1611 = call "DATA ENCRYPT STRING FILE WRITE.vi"("error in (no error)"=w2636, "User Action"="User Pressed Sway Right in MM", "main ref"=w2635) -> ("error out"=w2639:errorcluster)  [unwired: 6 in, 1 out]
        n1612 = call "SWAY WRITE FGV.vi"("Enum - Menu"=Sway_Write_enum."WRITE", "error in (no error)"=w2639, "main ref"=w2635) -> ("error out"=w2638:errorcluster)  [unwired: 8 in]
      }
      frame "Sway Right Main" {
        n1613 = call "Sway Right Main.vi"("error in (no error)"=w2648, "main ref"=w2646) -> ("error out"=w2647:errorcluster)  [unwired: 9 in]
        n1614 = Unbundle By Name(w2646) -> ("Platform Settings.Sway Right Main"=w2655:refnum<vi>)
        n1615 = property on="Property Node" class="Bool (strict)"(reference=w2655, "Value"=FALSE) -> (reference out=w2653:refnum<vi>, error out=w2654:errorcluster)  [unwired: 1 in]
        n1616 = Close Reference(reference=w2653, error in (no error)=w2654) -> ()  [unwired: 1 out]
        n1617 = call "DATA ENCRYPT STRING FILE WRITE.vi"("error in (no error)"=w2647, "User Action"="User Pressed Sway Right", "main ref"=w2646) -> ("error out"=w2650:errorcluster)  [unwired: 6 in, 1 out]
        n1618 = call "SWAY WRITE FGV.vi"("Enum - Menu"=Sway_Write_enum."WRITE", "error in (no error)"=w2650, "main ref"=w2646) -> ("error out"=w2649:errorcluster)  [unwired: 8 in]
      }
      frame "Manual Write Heave & Surge" {
        n1619 = Unbundle By Name(w2656) -> ("Heave AND Surge.Manual Write"=w2665:refnum<vi>)
        n1620 = property on="Property Node" class="Bool (strict)"(reference=w2665, "Value"=FALSE) -> (reference out=w2663:refnum<vi>, error out=w2664:errorcluster)  [unwired: 1 in]
        n1621 = Close Reference(reference=w2663, error in (no error)=w2664) -> ()  [unwired: 1 out]
        n1622 = call "DATA ENCRYPT STRING FILE WRITE.vi"("error in (no error)"=w2657, "User Action"="User Pressed Manual Write Heave and Surge", "main ref"=w2656) -> ("error out"=w2660:errorcluster)  [unwired: 6 in, 1 out]
        n1623 = call "HEAVE WRITE FGV.vi"("Enum - Menu"=Heave_Write_enum."WRITE", "error in (no error)"=w2660, "main ref"=w2656) -> ("error out"=w2659:errorcluster)  [unwired: 8 in]
      }
      frame "Manual Write SWAY" {
        n1624 = Unbundle By Name(w2667) -> ("SWAY.Manual Write SWAY"=w2675:refnum<vi>)
        n1625 = property on="Property Node" class="Bool (strict)"(reference=w2675, "Value"=FALSE) -> (reference out=w2673:refnum<vi>, error out=w2674:errorcluster)  [unwired: 1 in]
        n1626 = Close Reference(reference=w2673, error in (no error)=w2674) -> ()  [unwired: 1 out]
        n1627 = call "DATA ENCRYPT STRING FILE WRITE.vi"("error in (no error)"=w2668, "User Action"="User Pressed Manual Write Sway", "main ref"=w2667) -> ("error out"=w2670:errorcluster)  [unwired: 6 in, 1 out]
        n1628 = call "SWAY WRITE FGV.vi"("Enum - Menu"=Sway_Write_enum."WRITE", "error in (no error)"=w2670, "main ref"=w2667) -> ("error out"=w2669:errorcluster)  [unwired: 8 in]
      }
      frame "Manual Write TRACTION" {
        n1629 = Unbundle By Name(w2677) -> ("Traction.Manual Write TRACTION"=w2685:refnum<vi>)
        n1630 = property on="Property Node" class="Bool (strict)"(reference=w2685, "Value"=FALSE) -> (reference out=w2683:refnum<vi>, error out=w2684:errorcluster)  [unwired: 1 in]
        n1631 = Close Reference(reference=w2683, error in (no error)=w2684) -> ()  [unwired: 1 out]
        n1632 = call "DATA ENCRYPT STRING FILE WRITE.vi"("error in (no error)"=w2678, "User Action"="User Pressed Manual Write Traction", "main ref"=w2677) -> ("error out"=w2680:errorcluster)  [unwired: 6 in, 1 out]
        n1633 = call "TRACTION WRITE FGV.vi"("Enum - Menu"=Traction_Write_enum."WRITE", "error in (no error)"=w2680, "main ref"=w2677) -> ("error out"=w2679:errorcluster)  [unwired: 8 in]
      }
      frame "Manual Write ACQUOSTIC" {
        n1634 = local write "Manual Write Acquostic"(FALSE ("Manual Write Acquostic")) -> ()
        n1635 = call "DATA ENCRYPT STRING FILE WRITE.vi"("error in (no error)"=w2689, "User Action"="User Pressed Manual Write Acquostics", "main ref"=w2688) -> ("error out"=w2691:errorcluster)  [unwired: 6 in, 1 out]
        n1636 = call "Acq Write Loop.vi"("Enum - Menu"=Write_Main_Enum."WRITE", "error in (no error)"=w2691, "main ref"=w2688) -> ("error out"=w2690:errorcluster)  [unwired: 8 in]
      }
      frame "Load En" {
        # "zNL 2"
        n1637 = Unbundle By Name(w2694) -> ("Main Screen.Load En"=w2699:refnum<vi>)
        n1638 = property on="Property Node" class="Bool (strict)"(reference=w2699) -> (reference out=w2697:refnum<vi>, error out=w2698:errorcluster, "Value"=w2693:bool)  [unwired: 1 in]
        n1639 = Close Reference(reference=w2697, error in (no error)=w2698) -> ()  [unwired: 1 out]
        n1640 = case shown="False" w2693 {
          tunnel: [w2711 w2721] -> w2695
          tunnel: w2696 -> [w2713 w2720]
          tunnel: w2694 -> [w2701 w2715]
          tunnel: w2694 -> [w2709 _]
          tunnel: w2694 -> [w2708 _]
          frame False {
            n1641 = call "DATA ENCRYPT STRING FILE WRITE.vi"("error in (no error)"=w2713, "User Action"="User Pressed UnLoad on Main Screen", "main ref"=w2701) -> ("error out"=w2702:errorcluster)  [unwired: 6 in, 1 out]
            n1642 = call "Stall Data Flow.vim"("value in"=w2702, "milliseconds to wait"=u32 2000) -> ("value out"=w2707:errorcluster)  [unwired: 1 out]
            n1643 = Unbundle By Name(w2701) -> ("Main Screen.zNL 2"=w2705:refnum<vi>)
            n1644 = property on="Property Node" class="Bool (strict)"(reference=w2705, "DisabledEnum"=T31."Enabled" ("Disabled")) -> (reference out=w2703:refnum<vi>, error out=w2704:errorcluster)  [unwired: 1 in]
            n1645 = call "PID UNLOAD.vi"("error in (no error)"=w2707, "main ref"=w2708) -> ("error out"=w2710:errorcluster)  [unwired: 9 in]
            n1646 = Close Reference(reference=w2703, error in (no error)=w2704) -> ()  [unwired: 1 out]
            n1647 = call "HEAVE WRITE FGV.vi"("Enum - Menu"=Heave_Write_enum."WRITE", "error in (no error)"=w2710, "main ref"=w2709) -> ("error out"=w2711:errorcluster)  [unwired: 8 in]
          }
          frame True {
            n1648 = call "DATA ENCRYPT STRING FILE WRITE.vi"("error in (no error)"=w2720, "User Action"="User Pressed Load on Main Screen", "main ref"=w2715) -> ("error out"=w2721:errorcluster)  [unwired: 6 in, 1 out]
            n1649 = Unbundle By Name(w2715) -> ("Main Screen.zNL 2"=w2719:refnum<vi>)
            n1650 = property on="Property Node" class="Bool (strict)"(reference=w2719, "DisabledEnum"=T31."Disabled and Grayed Out" ("Disabled")) -> (reference out=w2717:refnum<vi>, error out=w2718:errorcluster)  [unwired: 1 in]
            n1651 = Close Reference(reference=w2717, error in (no error)=w2718) -> ()  [unwired: 1 out]
          }
        }
      }
      frame "apply load" {
        n1652 = Unbundle By Name(w2724) -> ("Main Screen.Load En"=w2729:refnum<vi>)
        n1653 = property on="Property Node" class="Bool (strict)"(reference=w2729) -> (reference out=w2727:refnum<vi>, error out=w2728:errorcluster, "Value"=w2723:bool)  [unwired: 1 in]
        n1654 = Close Reference(reference=w2727, error in (no error)=w2728) -> ()  [unwired: 1 out]
        n1655 = case shown="False" w2723 {
          tunnel: [w2736 w2743] -> w2725
          tunnel: w2726 -> [w2739 w2742]
          tunnel: w2724 -> [w2738 w2741]
          tunnel: w2724 -> [w2733 _]
          tunnel: w2724 -> [w2732 _]
          frame False {
            n1656 = call "DATA ENCRYPT STRING FILE WRITE.vi"("error in (no error)"=w2739, "User Action"="User Pressed UnLoad on Service Screen", "main ref"=w2738) -> ("error out"=w2735:errorcluster)  [unwired: 6 in, 1 out]
            n1657 = call "Stall Data Flow.vim"("value in"=w2735, "milliseconds to wait"=u32 2000) -> ("value out"=w2731:errorcluster)  [unwired: 1 out]
            n1658 = call "PID UNLOAD.vi"("error in (no error)"=w2731, "main ref"=w2732) -> ("error out"=w2734:errorcluster)  [unwired: 9 in]
            n1659 = call "HEAVE WRITE FGV.vi"("Enum - Menu"=Heave_Write_enum."WRITE", "error in (no error)"=w2734, "main ref"=w2733) -> ("error out"=w2736:errorcluster)  [unwired: 8 in]
          }
          frame True {
            n1660 = call "DATA ENCRYPT STRING FILE WRITE.vi"("error in (no error)"=w2742, "User Action"="User Pressed Load on Service Screen", "main ref"=w2741) -> ("error out"=w2743:errorcluster)  [unwired: 6 in, 1 out]
          }
        }
      }
      frame "BACK" {
        w2750 = FALSE ("Value")
        n1661 = Unbundle By Name(w2745) -> ("Main Screen.BACK"=w2770:refnum<vi>)
        n1662 = property on="Property Node" class="Bool (strict)"(reference=w2770, "Value"=FALSE) -> (reference out=w2768:refnum<vi>, error out=w2769:errorcluster)  [unwired: 1 in]
        n1663 = Close Reference(reference=w2768, error in (no error)=w2769) -> ()  [unwired: 1 out]
        n1664 = call "DATA ENCRYPT STRING FILE WRITE.vi"("error in (no error)"=w2767, "User Action"="User Pressed Back on Main Screen", "main ref"=w2745) -> ("error out"=w2765:errorcluster)  [unwired: 6 in, 1 out]
        n1665 = Unbundle By Name(w2745) -> ("Main Home Screen.MainPage"=w2757:refnum<vi>)
        n1666 = Unbundle By Name(w2745) -> ("Main Screen.Start Test"=w2753:refnum<vi>)
